vi "Set Target Heading.vi"(11 "Current Bearing":dbl) -> (3 "Target Heading":dbl)   [LabVIEW 2009]
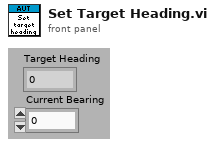
[diagram p1: front panel]
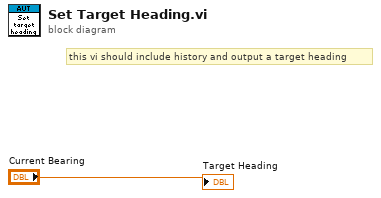
[diagram p0: block diagram]
diagram:
  # "this vi should include history and output a target heading"
  "Target Heading" <- "Current Bearing"
